vi "LS4 SetLimits.vi"(8 "error in (no error)":errorcluster, 10 "Axis":T1=1 items=["1"=1, "2"=2, "3"=3, "4"=4], 11 "DelayLineLS4 in":refnum<class "DLLS4.lvclass">) -> (0 "error out":errorcluster, 3 "DelayLineLS4 out":refnum<class "DLLS4.lvclass">)   [LabVIEW 2019, in "DLLS4.lvclass"]
uses:
  DLLS4.lvclass
  C:/Users/elysium/Documents/dev/TRANCON/Classes/Delay Line/DelayLine.lvclass
  C:/Users/elysium/Documents/dev/TRANCON/Classes/GeneralFunctionality/GeneralFunctionality.lvclass
  LS4 axis.ctl
  LS4_parameters.ctl
  DelayLine.lvclass/DelayLine.ctl
  GeneralFunctionality/GeneralFunctionality.lvclass/GeneralFunctionality.ctl
  <vilib>/Utility/error.llb/DialogType.ctl
  Config/Config.lvclass
  <vilib>/ErrorRing/Error Ring.xnode
  DelayLine.lvclass
  GeneralFunctionality/GeneralFunctionality.lvclass
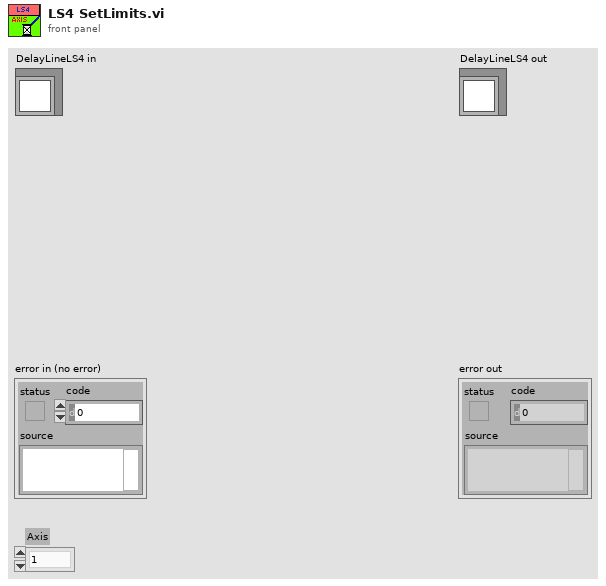
[diagram p1: front panel]
types:
  T1 = typedef "DelayLine.lvclass/LS4 axis.ctl" = u16
  T2 = typedef "DelayLine.lvclass/LS4_parameters.ctl" = string
  T3 = typedef "DialogType.ctl" = u16
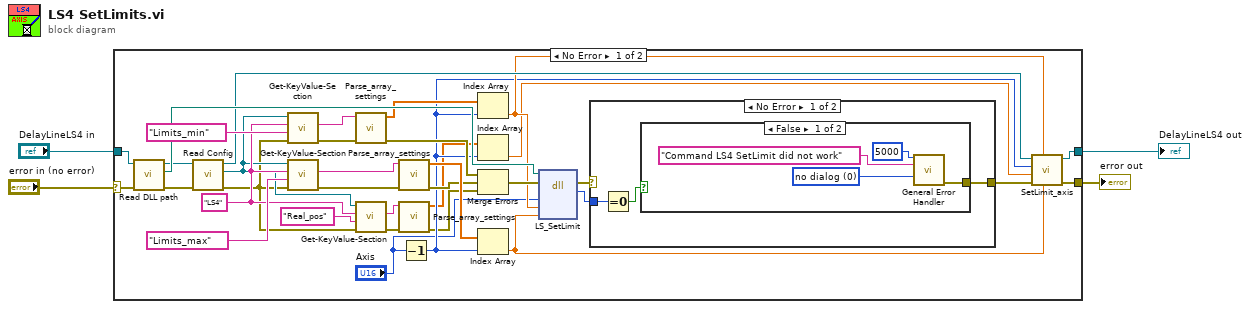
[diagram p0: block diagram]
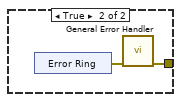
[diagram p2: hidden frame]
diagram:
  n1 = case shown="No Error" "error in (no error)" {
    selector: "error in (no error)" -> [w35 w51]
    tunnel: [w19 w52] -> w2
    tunnel: "DelayLineLS4 in" -> [w36 w52]
    tunnel: [w18 w51] -> w1
    frame No Error {
      w14 = "LS4" ("Section")
      n2 = call "Read DLL path.vi"("error in (no error)"=w35, "DelayLine in"=w36) -> ("error out"=w31:errorcluster, "DLL path"=w37:path, "DelayLine out"=w22:refnum<class "DLLS4.lvclass">)  [unwired: 7 in]
      n3 = call "Read Config.vi"("error in (no error)"=w31, "GeneralFunctionality en entrée"=w22) -> ("error out"=w12:errorcluster, "Config.lvclass"=w13:refnum<class "Config.lvclass">, "GeneralFunctionality en sortie"=w21:refnum<class "DLLS4.lvclass">)  [unwired: 7 in]
      n4 = call-dynamic "Get-KeyValue-Section.vi"("error in (no error)"=w12, "Key"=T2 "Limits_min" ("Section"), "Section"=w14, "Config in"=w13) -> ("error out"=w33:errorcluster, "Value"=w34:string)  [unwired: 5 in, 1 out]
      n5 = call-dynamic "Get-KeyValue-Section.vi"("error in (no error)"=w12, "Key"=T2 "Limits_max" ("Section"), "Section"=w14, "Config in"=w13) -> ("error out"=w29:errorcluster, "Value"=w28:string)  [unwired: 5 in, 1 out]
      n6 = call "Parse_array_settings.vi"("error in (no error)"=w33, "Value"=w34) -> ("error out"=w25:errorcluster, "Array"=w30:sgl[])  [unwired: 8 in]
      n7 = call-dynamic "Get-KeyValue-Section.vi"("error in (no error)"=w12, "Key"="Real_pos", "Section"=w14, "Config in"=w13) -> ("error out"=w8:errorcluster, "Value"=w9:string)  [unwired: 5 in, 1 out]
      n8 = call "Parse_array_settings.vi"("error in (no error)"=w29, "Value"=w28) -> ("error out"=w24:errorcluster, "Array"=w26:sgl[])  [unwired: 8 in]
      n9 = call "Parse_array_settings.vi"("error in (no error)"=w8, "Value"=w9) -> ("error out"=w7:errorcluster, "Array"=w10:sgl[])  [unwired: 8 in]
      n10 = Decrement(x="Axis") -> (x-1=w11:T1)
      n11 = Index Array(array=w30, index=w11) -> (element=w17:sgl)
      n12 = Index Array(array=w10, index=w11) -> (element=w6:sgl)
      n13 = Merge Errors(w25, w24, w7) -> (w23:errorcluster)
      n14 = Index Array(array=w26, index=w11) -> (element=w16:sgl)
      n15 = dll-call lib="LStep4.dll" fn="LS_SetLimit"(path in=w37, error in=w23, "Axis"="Axis", "MinRange"=w17, "MaxRange"=w16) -> (error out=w39:errorcluster, "type de retour"=w38:i32)  [unwired: 4 in, 1 out]
      n16 = case shown="No Error" w39 {
        selector: w39 -> [_ w50]
        tunnel: w38 -> [w42 _]
        tunnel: [w41 w50] -> w20
        frame No Error {
          n17 = Equal To 0?(x=w42) -> (x = 0?=w40:bool)
          n18 = case shown="False" w40 {
            tunnel: [w44 w47] -> w41
            frame False {
              w43 = T3 0 items=["no dialog", "OK message", "continue or stop message", "OK message + warnings", "continue/stop + warnings"] ("type of dialog (OK msg:1)")
              n19 = call <vilib>:"General Error Handler.vi"("[error code] (0)"=5000 ("code"), "[error source] (\" \")"="Command LS4 SetLimit did not work" ("String to Prepend to source (\"\")"), "type of dialog (OK msg:1)"=w43) -> ("error out"=w44:errorcluster)  [unwired: 8 in, 4 out]
            }
            frame True {
              n20 = xnode "Error Ring"() -> ("error out"=w48:errorcluster)
              n21 = call <vilib>:"General Error Handler.vi"("error in (no error)"=w48) -> ("error out"=w47:errorcluster)  [unwired: 10 in, 4 out]
            }
          }
        }
        frame Error {
        }
      }
      n22 = call-dynamic "SetLimit_axis.vi"("max"=w16, "min"=w17, "error in (no error)"=w20, "real pos zero"=w6, "Axis"=w11, "DelayLine in"=w21) -> ("error out"=w18:errorcluster, "DelayLine out"=w19:refnum<class "DLLS4.lvclass">)  [unwired: 4 in]
    }
    frame Error {
    }
  }
  "error out" <- w1
  "DelayLineLS4 out" <- w2
